vi "uTTA_SendQuery.vi"(4 "RX Termination(\\n)":string="\n", 6 "Timeout(ms)":i32=1000, 7 "Send String":string, 8 "error in (no error)":errorcluster, 10 "TX Termination(\\n)":string="\n", 11 "VISA Refnum in":refnum<visa-resource-name>) -> (0 "error out":errorcluster, 2 "Received":string, 3 "VISA Refnum out":refnum<visa-resource-name>)   [LabVIEW 2021]
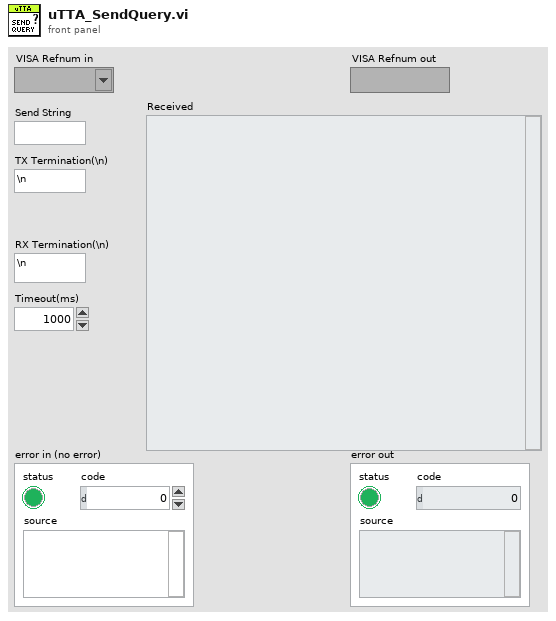
[diagram p1: front panel]
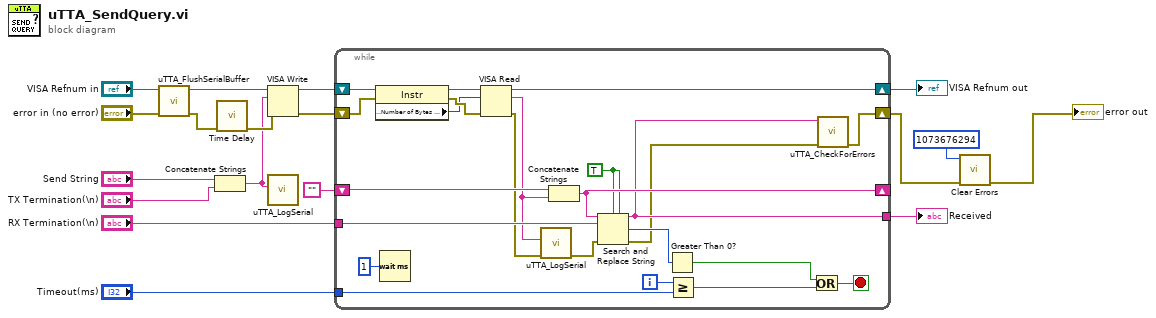
[diagram p0: block diagram]
diagram:
  n1 = call "uTTA_FlushSerialBuffer.vi"("error in (no error)"="error in (no error)", "VISA Refnum in"="VISA Refnum in") -> ("error out"=w1:errorcluster, "VISA Refnum out"=w2:refnum<visa-resource-name>)  [unwired: 4 in]
  n2 = Concatenate Strings("Send String", "TX Termination(\\n)") -> (w5:string)
  n3 = call "Time Delay"("error in (no error)"=w1) -> ("error out"=w8:errorcluster)  [unwired: 10 in]
  n4 = VISA Write(VISA resource name=w2, write buffer=w5, error in (no error)=w8) -> (VISA resource name out=w12:refnum<visa-resource-name>, error out=w13:errorcluster)  [unwired: 1 out]
  n5 = call "uTTA_LogSerial.vi"("Data_Sent"=w5) -> ()  [unwired: 6 in, 1 out]
  n6 = while {
    shift-right: [w35] -> _
    shift-left: "" -> [w36]
    tunnel: [w25] -> w7
    shift-right: [w23] -> w10
    shift-left: w13 -> [w40]
    shift-right: [w32] -> w17
    shift-left: w12 -> [w41]
    tunnel: "Timeout(ms)" -> [w27]
    tunnel: "RX Termination(\\n)" -> [w26]
    i -> [w28]
    stop <- w30 stop-if-true
    w22 = TRUE ("ignore case? (F)")
    n7 = property class="Instr"(reference=w41, error in=w40) -> (reference out=w39:refnum<visa-resource-name>, error out=w38:errorcluster, "Serial Settings:Number of Bytes at Serial Port"=w37:u32)
    n8 = Wait (ms)(milliseconds to wait=u32 1) -> ()  [unwired: 1 out]
    n9 = VISA Read(VISA resource name=w39, byte count=w37, error in (no error)=w38) -> (VISA resource name out=w32:refnum<visa-resource-name>, read buffer=w21:string, error out=w20:errorcluster)  [unwired: 1 out]
    n10 = call "uTTA_LogSerial.vi"("error in"=w20, "Data_Sent"=w21) -> ("error out"=w19:errorcluster)  [unwired: 5 in]
    n11 = Concatenate Strings(w36, w21) -> (w35:string)
    n12 = Search and Replace String(case sensitive?=w22, multiline?=w22, input string=w35, search string=w26, error in=w19) -> (result string=w25:string, number of replacements=w34:i32, error out=w24:errorcluster)  [unwired: 3 in, 1 out]
    n13 = Greater Than 0?(x=w34) -> (x > 0?=w31:bool)
    n14 = Greater Or Equal?(x=w28, y=w27) -> (x >= y?=w29:bool)
    n15 = Or(x=w31, y=w29) -> (x .or. y?=w30:bool)
    n16 = call "uTTA_CheckForErrors.vi"("error in"=w24, "Received"=w25) -> ("error out"=w23:errorcluster)  [unwired: 9 in]
  }
  "Received" <- w7
  "VISA Refnum out" <- w17
  n17 = call <vilib>:"Clear Errors.vi"("error in (no error)"=w10, "specific error code to clear (0: all)"=1073676294) -> ("error out"=→"error out":errorcluster)  [unwired: 4 in, 1 out]
